vi "Build_Read Discrete Inputs.vi"(8 "error in (no error)":errorcluster, 9 "quantity":u16, 10 "starting address":u16) -> (0 "error out":errorcluster, 3 "MB_PDU":T1={"Function Code"=1, "Data"=[], "RTU_DataBytes"=0})   [LabVIEW 2021, in "MB Master.lvlib"]
doc: "Builds PDU for Read Discrete Inputs (function code 2)."
uses:
  <vilib>/Plasmionique/MB Master/MB Master.lvlib
  <vilib>/Plasmionique/MB Master/MB_PDU/MB_PDU_Cluster.ctl
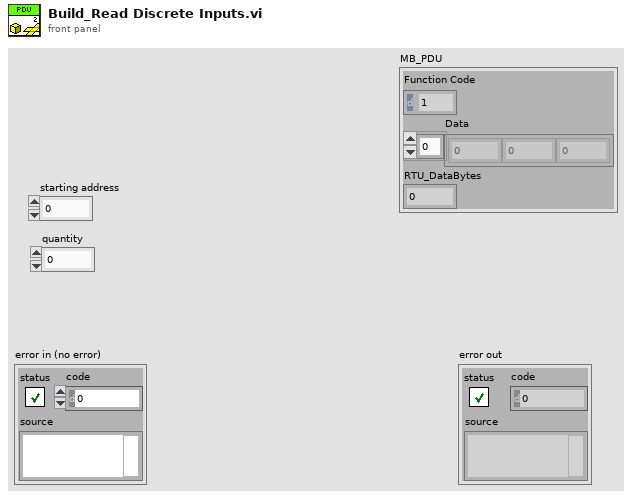
[diagram p1: front panel]
types:
  T1 = typedef "MB Master.lvlib/MB_PDU_Cluster.ctl" = cluster{"Function Code":u8, "Data":u8[], "RTU_DataBytes":i32}
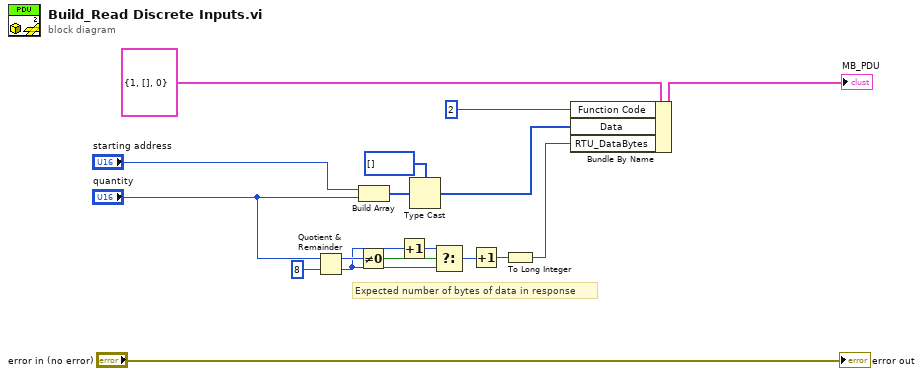
[diagram p0: block diagram]
diagram:
  # "Expected number of bytes of data in response"
  n1 = Quotient & Remainder(x="quantity", y=u16 8) -> (x-y*floor(x/y)=w8:u16, floor(x/y)=w5:u16)
  n2 = Not Equal To 0?(x=w8) -> (x != 0?=w7:bool)
  n3 = Build Array("starting address", "quantity") -> (w17:u16[])
  n4 = Increment(x=w5) -> (x+1=w6:u16)
  n5 = Type Cast(type=u8[] [], x=w17) -> (*(type *) &x=w12:u8[])
  n6 = Select(t=w6, s=w7, f=w5) -> (s? t:f=w4:u16)
  n7 = Increment(x=w4) -> (x+1=w3:u16)
  n8 = To Long Integer(number=w3) -> (32bit integer=w1:i32)
  n9 = Bundle By Name(cluster=T1 {"Function Code"=1, "Data"=[], "RTU_DataBytes"=0} ("Modbus Serial New.lvlib:MB_PDU.lvclass"), "Function Code"=u8 2, "Data"=w12, "RTU_DataBytes"=w1) -> (→"MB_PDU":T1)
  "error out" <- "error in (no error)"
